vi "CRYGet Custom VIs.vi"(11 "Category":string="stimulus.txt") -> (3 "Custom VI Editor Names":string[](array[string]))   [LabVIEW 2013]
uses:
  CRYMainGlobal.vi
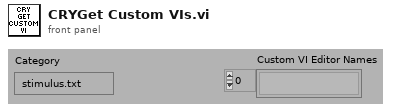
[diagram p1: front panel]
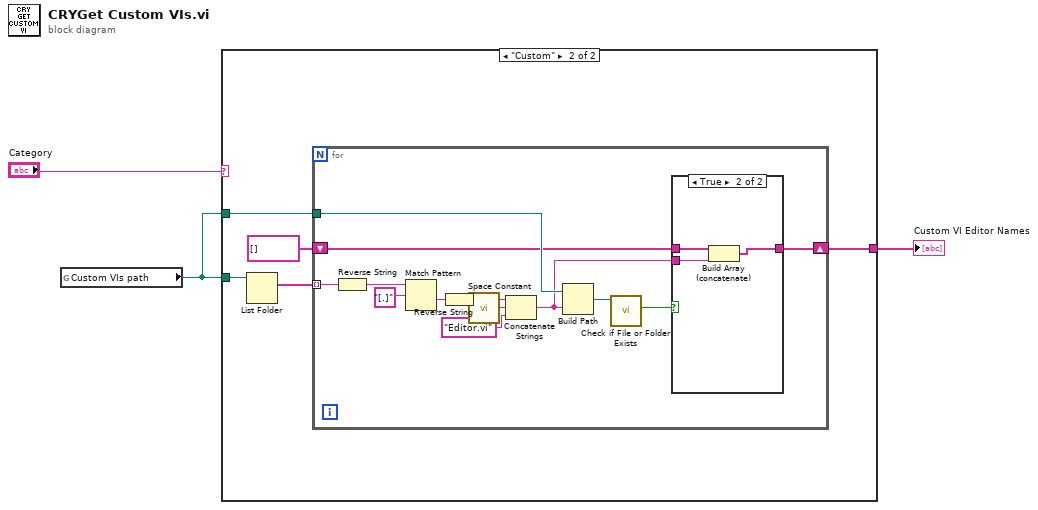
[diagram p0: block diagram]
diagram:
  n1 = global read "CRYMainGlobal.vi" "Custom VIs path"() -> (w2:path)
  n2 = case shown="\"Custom\"" "Category" {
    tunnel: w2 -> [_ w8]
    tunnel: w2 -> [_ w5]
    tunnel: [_ w4] -> w1
    frame Default {
    }
    frame "Custom" {
      n3 = List Folder(path=w8) -> (filenames=w7:string[])  [unwired: 1 in, 5 out]
      n4 = for {
        tunnel: w7 -> [w10] mode=indexing
        shift-right: [w11] -> w4
        shift-left: string[] [] ("filenames") -> [w12]
        tunnel: w5 -> [w15]
        n5 = Reverse String(1:w10) -> (0:w19:string)
        n6 = Match Pattern(string=w19, regular expression="[.]") -> (after substring=w20:string)  [unwired: 4 out]
        n7 = Reverse String(1:w20) -> (0:w13:string)
        n8 = call <vilib>:"Space Constant.vi"() -> ("String"=w17:string)
        n9 = Concatenate Strings(w13, w17, "Editor.vi" ("string")) -> (w9:string)
        n10 = Build Path(base path=w15, name or relative path=w9) -> (appended path=w16:path)
        n11 = call <vilib>:"Check if File or Folder Exists.vi"("path"=w16) -> ("file or folder exists?"=w14:bool)  [unwired: 8 in, 2 out]
        n12 = case shown="True" w14 {
          tunnel: w9 -> [_ w24]
          tunnel: w12 -> [w22 w25]
          tunnel: [w22 w23] -> w11
          frame False {
          }
          frame True {
            n13 = Build Array (concatenate)(w25, w24) -> (w23:string[])
          }
        }
      }
    }
  }
  "Custom VI Editor Names" <- w1
